vi "4000_Module_configure.vi"() -> ()   [LabVIEW 2010]
panel:
  in  "Individual Input Ranges":bool
  in  "Port Name":string="MainNetwork"
  in  "Use checksum":bool caption="Checksum Required to configure?"
  in  "Range Setting":u16(ring)=15 items=["00     +/-15mV", "01     +/-50mV", "02     +/-100mV", "03     +/-500mV", "04     +/-1V", "05     +/-2.5V", "06     +/-20mA", "NOT USED", "08     +/-10V", "09     +/-5V", "0A     +/-1V", "0B     +/-500mV", "0C     +/-150mV", "0D     +/-20mA", "0E     Type J", "0F     Type K", "10     Type T", "11     Type E", "12     Type R", "13     Type S", "14     Type B"]
  in  "Baud Rate (9600)":u16(ring)=3 items=["1200 bps", "2400 bps", "4800 bps", "9600 bps", "19.2 kbps", "38.4 kbps"]
  in  "Data Format":u16(ring) items=["Engineering Units", "% of FSR", "Hex", "Ohms (4013)"]
  in  "Mains Frequency":bool=TRUE
  out "Reply":string
  in  "Cheksum":bool=TRUE
  out "String Sent":string
  in  "New Address":u8
  in  "Old Address":u8
  # "Happy reply starts \"!\"\nUnhappy reply starts \"?\""
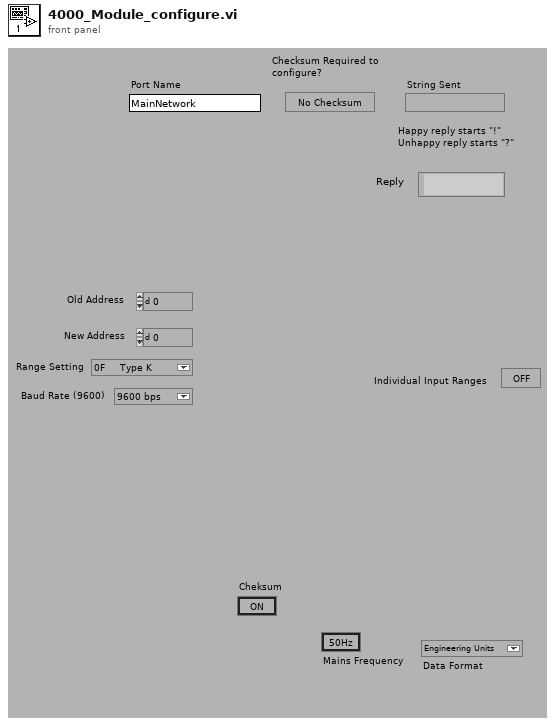
[diagram p1: front panel]
types:
  T1 = cluster{"Boolean array[0]":bool, "Boolean array[1]":bool}
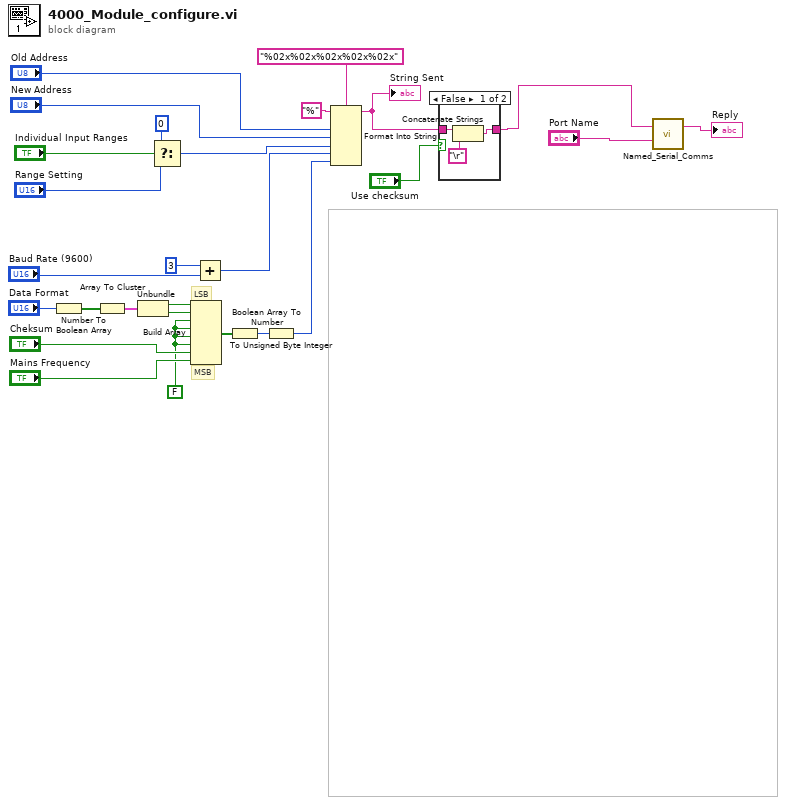
[diagram p0: block diagram]
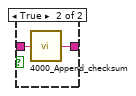
[diagram p2: hidden frame]
diagram:
  w17 = FALSE
  # "MSB"
  # "LSB"
  n1 = Number To Boolean Array(number="Data Format") -> (Boolean array=w15:bool[])
  n2 = Array To Cluster(array=w15) -> (cluster=w14:T1)
  n3 = Unbundle(w14) -> ("Boolean array[0]"=w13:bool, "Boolean array[1]"=w12:bool)
  n4 = Select(t=u16 0, s="Individual Input Ranges", f="Range Setting") -> (s? t:f=w4:u16)
  n5 = Build Array(w13, w12, w17, w17, w17, w17, "Cheksum", "Mains Frequency") -> (w23:bool[])
  n6 = Add(x=u16 3, y="Baud Rate (9600)") -> (x+y=w10:u16)
  n7 = Boolean Array To Number(Boolean array=w23) -> (number=w21:u32)
  n8 = To Unsigned Byte Integer(number=w21) -> (unsigned 8bit integer=w20:u8)
  n9 = Format Into String(format string="%02x%02x%02x%02x%02x", initial string="%", "Old Address", "New Address", w4, w10, w20) -> (resulting string=w19:string)  [unwired: 1 in, 1 out]
  "String Sent" <- w19
  n10 = case shown="False" "Use checksum" {
    tunnel: w19 -> [w30 w32]
    tunnel: [w29 w31] -> w6
    frame False {
      n11 = Concatenate Strings(w30, "\r") -> (w29:string)
    }
    frame True {
      n12 = call "4000_Append_checksum.vi"("ADAM command"=w32) -> ("ADAM string to send"=w31:string)
    }
  }
  n13 = call "Named_Serial_Comms.vi"("Write String"=w6, "Port Name"="Port Name") -> ("Read"=→"Reply":string)  [unwired: 10 in, 3 out]
